vi "Query Timestamp.vi"(8 "error in (no error)":errorcluster, 11 "VISA resource name":refnum<visa-resource-name>) -> (0 "error out":errorcluster, 2 "Timestamp":string, 3 "VISA resource name out":refnum<visa-resource-name>)   [LabVIEW 2020, in "Rohde&Schwarz CMXP Base.lvlib"]
doc: "This command queries a timestamp with the current system time. A query returns seven values, separated by commas:\nYear, month, day, hour, minutes, seconds, milliseconds\n\nAttribute:\nRSCMXPBASE_ATTR_QUERY_TIMESTAMP\n\nRemote-control command:\nSYSTem:TIME:HRTimer:ABSolute:SET?"
uses:
  <instrlib>/Rohde&Schwarz CMXP Base/Rohde&Schwarz CMXP Base.lvlib
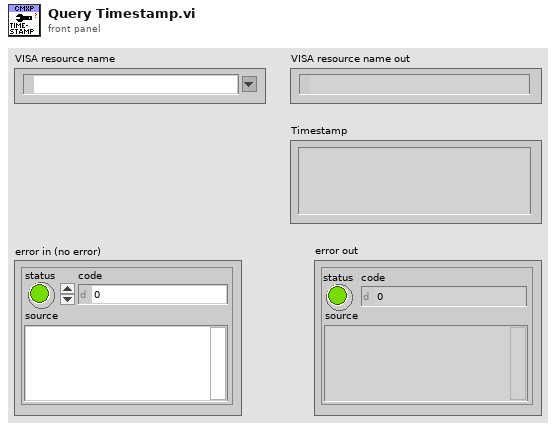
[diagram p1: front panel]
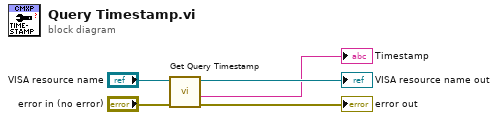
[diagram p0: block diagram]
diagram:
  n1 = call "Get Query Timestamp"("error in (no error)"="error in (no error)", "instrument handle"="VISA resource name") -> ("error out"=→"error out":errorcluster, "Query Timestamp"=→"Timestamp":string, "instrument handle out"=→"VISA resource name out":refnum<visa-resource-name>)  [unwired: 7 in]
